vi "RegistersRead.vi"(8 "error out":errorcluster) -> (0 "error out":errorcluster, 4 "Registers Init Value":u32[](array[numeric])=[3413, 6655, 32767, 32767, 16384, 160, 6656])   [LabVIEW 2012]
uses:
  <vilib>/Utility/NIReport.llb/NI_report.lvclass
  <vilib>/Utility/NIReport.llb/HTML/NI_HTML.lvclass
panel:
  in  "Instrument VISA in":T1={"AWG VISA"="AgilentGenerator1", "Oscilloscope  VISA "="AgilentOsciloscope", "Integration Board IP"="172.16.17.48", "connection ID"=refnum, "report out"=refnum, "report file path"=path "C:/Documents and Settings/CTA_LAB01/Desktop/L0_Asic/L0 Asic Test Data"}
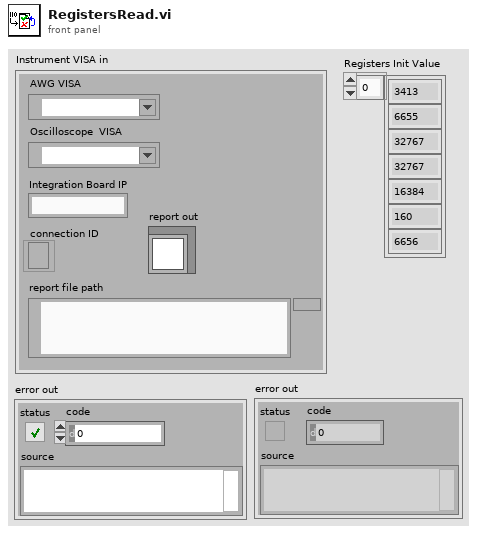
[diagram p1: front panel]
types:
  T1 = cluster{"AWG VISA":refnum<visa-resource-name>, "Oscilloscope  VISA ":refnum<visa-resource-name>, "Integration Board IP":string, "connection ID":refnum<k5>, "report out":refnum<class "NI_report.lvclass">, "report file path":path}
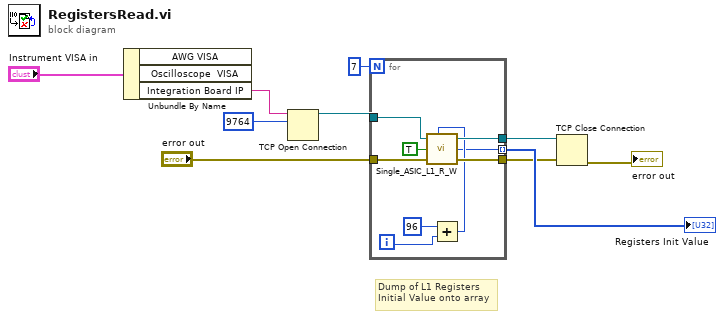
[diagram p0: block diagram]
diagram:
  # "Dump of L1 Registers\nInitial Value onto array"
  n1 = Unbundle By Name("Instrument VISA in") -> ("Integration Board IP"=w6:string)  [unwired: 2 out]
  n2 = TCP Open Connection(address=w6, remote port or service name=9764) -> (connection ID=w4:refnum<k5>)  [unwired: 3 in, 1 out]
  n3 = for {
    N: 7 -> [_]
    tunnel: "error out" -> [w19]
    tunnel: [w18] -> w2
    tunnel: w4 -> [w17]
    tunnel: [w15] -> w3
    tunnel: [w11] -> w10 mode=indexing
    i -> [w13]
    n4 = Add(x=96 ("y"), y=w13) -> (x+y=w12:i32)
    n5 = call "Single_ASIC_L1_R_W.vi"("connection ID"=w17, "Register or channel"=w12, "RD/#WR"=TRUE, "error in (no error)"=w19) -> ("connection ID out"=w15:refnum<k5>, "data read value"=w11:i64, "error out"=w18:errorcluster)  [unwired: 2 in, 1 out]
  }
  "Registers Init Value" <- w10
  n6 = TCP Close Connection(connection ID=w3, error in (no error)=w2) -> (error out=→"error out":errorcluster)  [unwired: 1 in, 1 out]
